vi "CFN61G_U8-to-B84-86_v1.vi"(11 "U8_Input":u8[](array[numeric])) -> (0 "Status_Word_Byte":bool[](array[boolean]), 1 "BIT_Status_Word":u16, 2 "DV_Byte":u8, 3 "Data_Validity_Byte":bool[](array[boolean]))   [LabVIEW 2017]
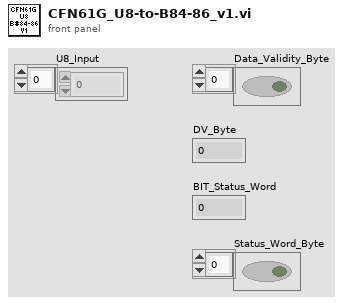
[diagram p1: front panel]
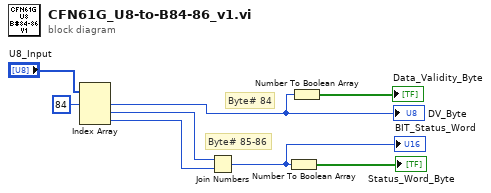
[diagram p0: block diagram]
diagram:
  # "Byte# 85-86"
  # "Byte# 84"
  n1 = Index Array(array="U8_Input", index #1=84 ("index")) -> (element #1=w6:u8, element #2=w7:u8, element #3=w8:u8)  [unwired: 2 in]
  "DV_Byte" <- w6
  n2 = Join Numbers(hi=w7, lo=w8) -> ((hi.lo)=w3:u16)
  "BIT_Status_Word" <- w3
  n3 = Number To Boolean Array(number=w3) -> (Boolean array=→"Status_Word_Byte":bool[])
  n4 = Number To Boolean Array(number=w6) -> (Boolean array=→"Data_Validity_Byte":bool[])
